vi "Sample_SimpleCoEWrite.vi"() -> ()   [LabVIEW 2022 SP3, in "EtherCAT_Library.lvlib"]
uses:
  EtherCAT_Library.lvlib
panel:
  out "error out":errorcluster
  in  "error in (no error)":errorcluster
  in  "Data":u8[](array[numeric]) format="%x"
  in  "SubIndex":u8=1 format="%x"
  in  "Index":u16=64256 format="%x"
  in  "Device address":string="192.168.80.50.4.1:1009"
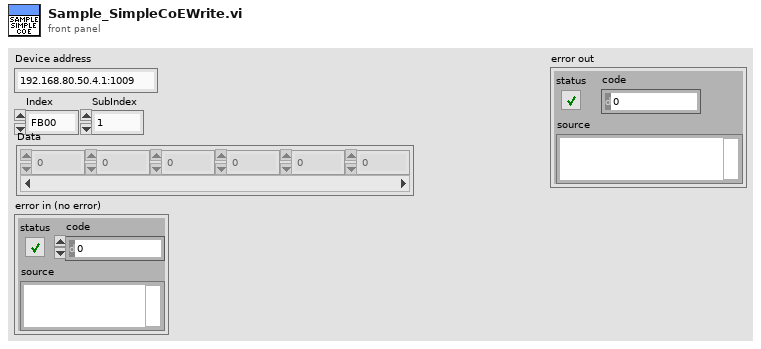
[diagram p1: front panel]
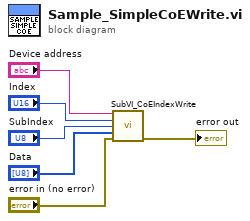
[diagram p0: block diagram]
diagram:
  n1 = call "SubVI_CoEIndexWrite.vi"("Device address"="Device address", "Index"="Index", "SubIndex"="SubIndex", "Data"="Data", "error in (no error)"="error in (no error)") -> ("error out"=→"error out":errorcluster)  [unwired: 10 in]
